vi "ScreenShake.vi"(8 "error in (no error)":errorcluster, 9 "Magnitude(5)":dbl=5.0, 10 "Duration(0,1)":dbl=0.1) -> (0 "error out":errorcluster)   [LabVIEW 2019, in "RT_Game.lvlib" / "Engine.lvclass"]
uses:
  Engine.lvclass
  MessageCluster.ctl
  ShakeMessageData.ctl
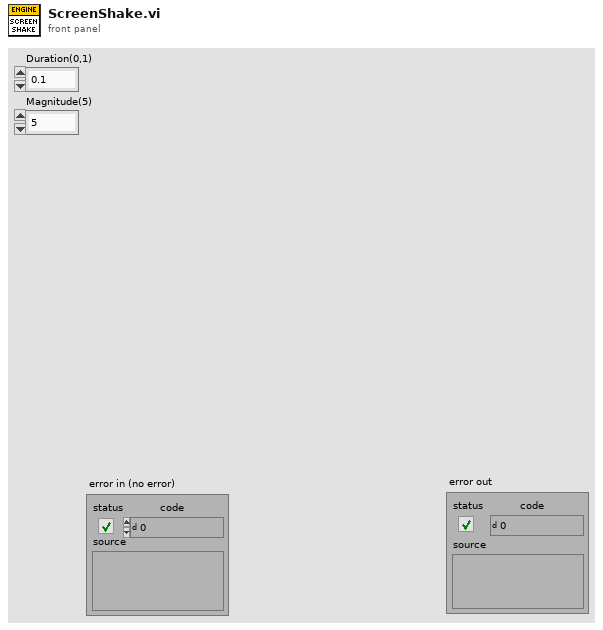
[diagram p1: front panel]
types:
  T1 = typedef "RT_Game.lvlib/Engine.lvclass/ShakeMessageData.ctl" = cluster{"Duration":dbl, "Magnitude":dbl}
  T2 = typedef "RT_Game.lvlib/Engine.lvclass/MessageCluster.ctl" = cluster{"Message":string, "Data":variant}
  T3 = typedef "RT_Game.lvlib/Engine.lvclass/Queues.ctl" = cluster{"MusicQueue":refnum<queue>, "TilesQueue":refnum<queue>, "SoundsQueue":refnum<queue>}
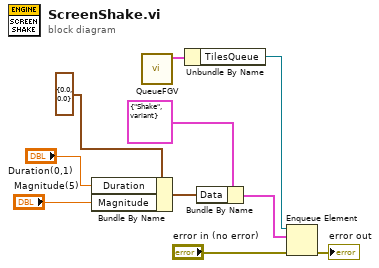
[diagram p0: block diagram]
diagram:
  n1 = Bundle By Name(cluster=T1 {"Duration"=0.0, "Magnitude"=0.0} ("ShakeMessageData"), "Duration"="Duration(0,1)", "Magnitude"="Magnitude(5)") -> (w3:T1)
  n2 = call "QueueFGV.vi"() -> ("Queues out"=w8:T3)  [unwired: 10 in, 1 out]
  n3 = Unbundle By Name(w8) -> ("TilesQueue"=w7:refnum<queue>)
  n4 = Bundle By Name(cluster=T2 {"Message"="Shake", "Data"=variant} ("element"), "Data"=w3) -> (w5:T2)
  n5 = Enqueue Element(queue=w7, element=w5, error in (no error)="error in (no error)") -> (error out=→"error out":errorcluster)  [unwired: 1 in, 2 out]
